vi "label_binarize.vi"(8 "error in":errorcluster caption="entrée d'erreur", 10 "y":string[][](array[string]), 11 "label_binarize":T2={"classes"=[], "neg_label"=0, "pos_label"=1, "sparse_output"=FALSE}) -> (0 "error out":errorcluster caption="sortie d'erreur", 3 "Data":T1)   [LabVIEW 2020]
doc: "Binarize labels in a one-vs-all fashion\n\nSeveral regression and binary classification algorithms are available in scikit-learn. A simple way to extend these algorithms to the multi-class classification case is to use the so-called one-vs-all scheme.\n\nThis function makes it possible to compute this transformation for a fixed set of class labels known ahead of time.\n\nParameters : \n\n- y : array-like\nSequence of integer labels or multilabel data to encode.\n\n- classes : array-like of shape [n_classes]\nUniquely holds the label for each class.\n\n- neg_label : int (default: 0)\nValue with which negative labels must be encoded.\n\n- pos_label : int (default: 1)\nValue with which positive labels must be encoded.\n\n- sparse_output : boolean (default: False),\nSet to true if output binary array is desired in CSR sparse format\n\nReturns : \n\n- Y : numpy array or CSR matrix of shape [n_samples, n_classes]\nShape will be [n_samples, 1] for binary problems."
uses:
  label_binarize.lvclass
panel:
  out "label_binarize.lvclass":refnum<class "label_binarize.lvclass">
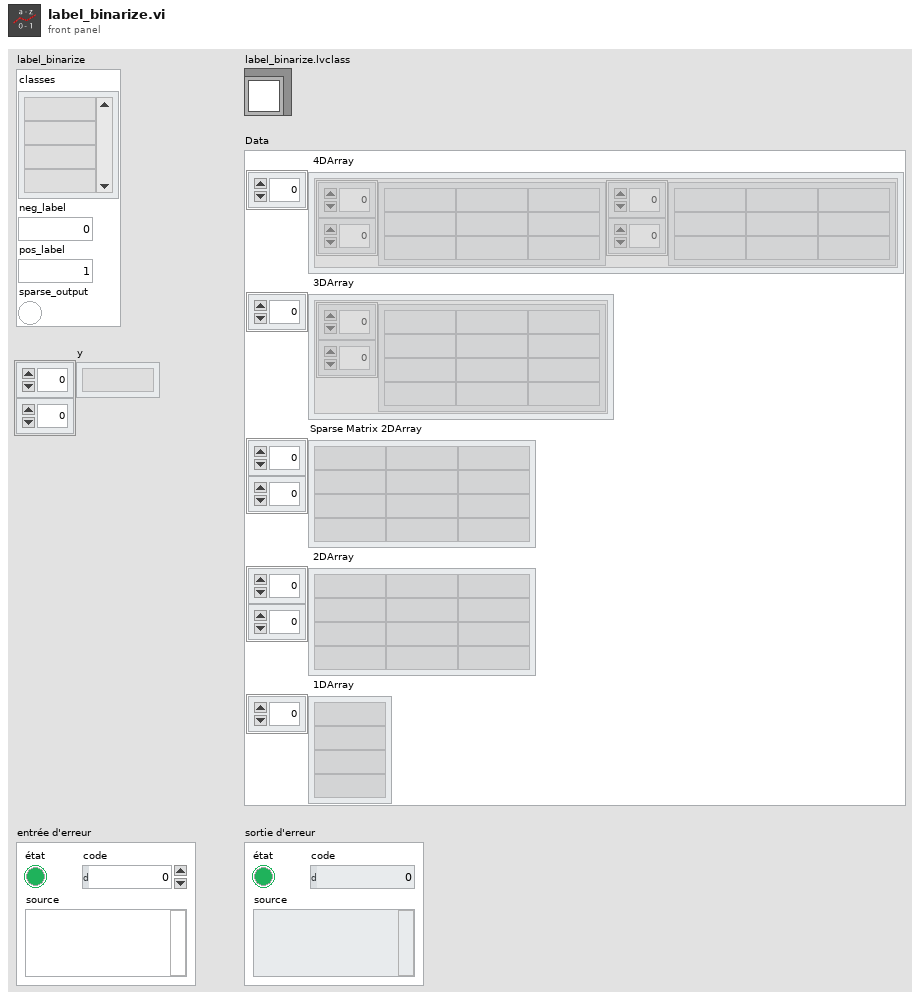
[diagram p1: front panel]
types:
  T1 = cluster{" 4DArray":cluster{"1":string[][], "2":string[][]}[], " 3DArray":cluster{"Tableau":string[][]}[], "Sparse Matrix 2DArray":string[][], " 2DArray":string[][], " 1DArray":string[]}
  T2 = cluster{"classes":string[][], "neg_label":i32, "pos_label":i32, "sparse_output":bool}
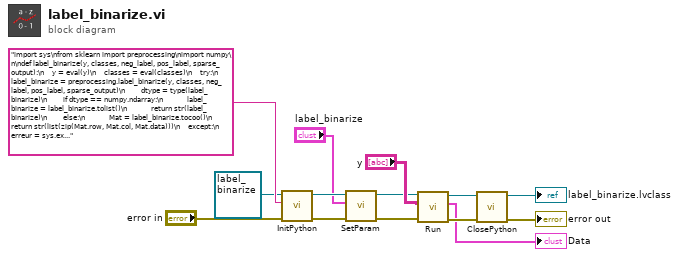
[diagram p0: block diagram]
diagram:
  n1 = call-dynamic "InitPython.vi"("error in (no error)"="error in", "Python Instruction"="import sys\nfrom sklearn import preprocessing\nimport numpy\n\ndef label_binarize(y, classes, neg_label, pos_label, sparse_output):\n    y = eval(y)\n    classes = eval(classes)\n    try:\n        label_binarize = preprocessing.label_binarize(y, classes, neg_label, pos_label, sparse_output)\n        dtype = type(label_binarize)\n        if dtype == numpy.ndarray:\n            label_binarize = label_binarize.tolist()\n            return str(label_binarize)\n        else:\n            Mat = label_binarize.tocoo()\n            return str(list(zip(Mat.row, Mat.col, Mat.data)))\n    except:\n        erreur = sys.exc_info()\n        typerr = u\"%s\" % (erreur[0])\n        typerr = typerr[typerr.find(\"'\")+1:typerr.rfind(\"'\")]\n        msgerr = u\"%s\" % (erreur[1])\n        message = str('/!\\\\ {0} : {1}'. format(typerr,msgerr))\n        return message", "Scikit-learn en entrée"=refnum<class "label_binarize.lvclass"> refnum ("label_binarize.lvclass")) -> ("error out"=w8:errorcluster, "Scikit-learn en sortie"=w10:refnum<class "label_binarize.lvclass">)  [unwired: 7 in]
  n2 = call-dynamic "SetParam.vi"("error in (no error)"=w8, "label_binarize"="label_binarize", "label_binarize.lvclass"=w10) -> ("error out"=w5:errorcluster, "label_binarize.lvclass"=w6:refnum<class "label_binarize.lvclass">)  [unwired: 7 in]
  n3 = call-dynamic "Run.vi"("error in (no error)"=w5, "y"="y", "label_binarize.lvclass"=w6) -> ("error out"=w3:errorcluster, "Data"=→"Data":T1, "label_binarize.lvclass"=w4:refnum<class "label_binarize.lvclass">)  [unwired: 6 in]
  n4 = call-dynamic "ClosePython.vi"("error in (no error)"=w3, "Scikit-learn en entrée"=w4) -> ("error out"=→"error out":errorcluster, "Scikit-learn en sortie"=→"label_binarize.lvclass":refnum<class "label_binarize.lvclass">)  [unwired: 8 in]
